vi "Post Iterate.vi"(8 "error in (no error)":errorcluster, 11 "Example Actor in":refnum<class "Example Actor.lvclass">) -> (0 "error out":errorcluster, 3 "Example Actor out":refnum<class "Example Actor.lvclass">)   [LabVIEW 2021, in "Example Iterator NR Actor Explicit Iteration.lvlib" / "Example Actor.lvclass"]
doc: "Method called after the iterations"
uses:
  Example Actor.lvclass
  Example Actor.lvclass/Example Actor.ctl
  Iterator NR Actor/Iterator NR Actor Messages/Notify Iteration Msg/Notify Iteration Msg.lvclass
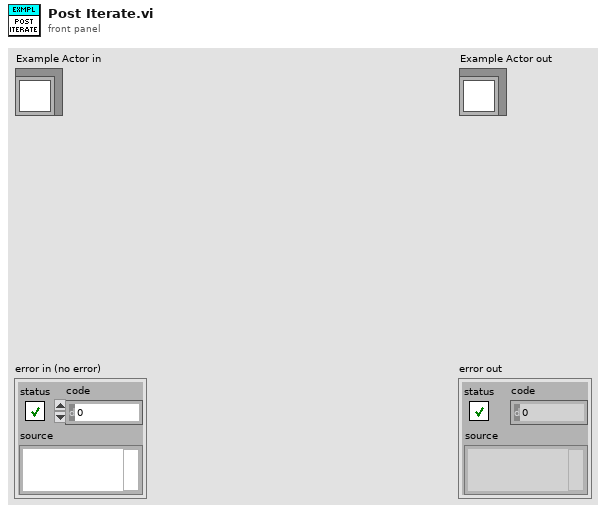
[diagram p1: front panel]
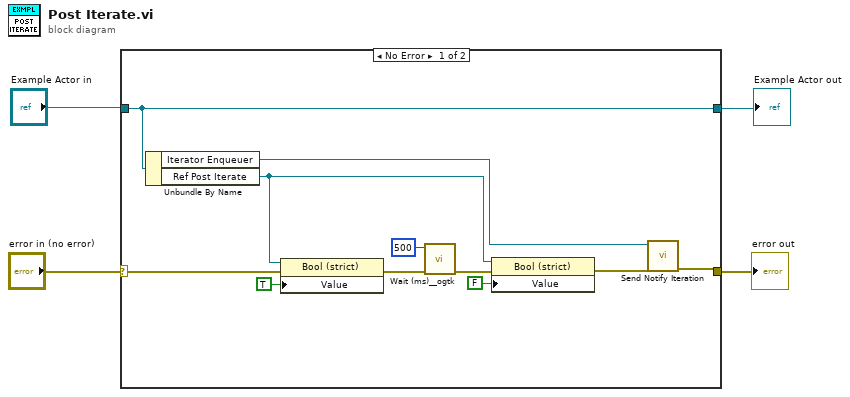
[diagram p0: block diagram]
diagram:
  n1 = case shown="No Error" "error in (no error)" {
    selector: "error in (no error)" -> [w14 w17]
    tunnel: [w6 w17] -> w1
    tunnel: [w15 w16] -> w3
    tunnel: "Example Actor in" -> [w15 w16]
    frame No Error {
      n2 = Unbundle By Name(w15) -> ("Iterator Enqueuer"=w5:refnum<class "Message Enqueuer.lvclass">, "Ref Post Iterate"=w11:refnum<vi>)
      n3 = property class="Bool (strict)"(reference=w11, error in=w14, "Value"=TRUE) -> (error out=w13:errorcluster)  [unwired: 1 out]
      n4 = call <userlib>:"Wait (ms)__ogtk.vi"("error in (no error)"=w13, "milliseconds to wait"=u32 500) -> ("error out"=w12:errorcluster)  [unwired: 8 in, 1 out]
      n5 = property class="Bool (strict)"(reference=w11, error in=w12, "Value"=FALSE) -> (error out=w7:errorcluster)  [unwired: 1 out]
      n6 = call "Send Notify Iteration.vi"("error in (no error)"=w7, "Message Enqueuer in"=w5) -> ("error out"=w6:errorcluster)  [unwired: 8 in, 1 out]
    }
    frame Error {
    }
  }
  "error out" <- w1
  "Example Actor out" <- w3
